vi "ReadBuffer.vi"(2 "Data type":T1(ring)=enum."I16", 5 "Pointer and BufferSize":u64[](array[numeric]), 7 "Offset":u64, 9 "Buffer size":i32, 11 "error in (no error)":errorcluster) -> (6 "Output Array":i16[](array[numeric]), 15 "error out":errorcluster)   [LabVIEW 2020]
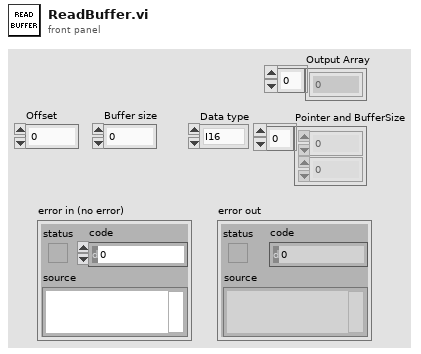
[diagram p1: front panel]
types:
  T1 = enum16{"U8", "I8", "U16", "I16", "U32", "I32", "U64", "I64"}
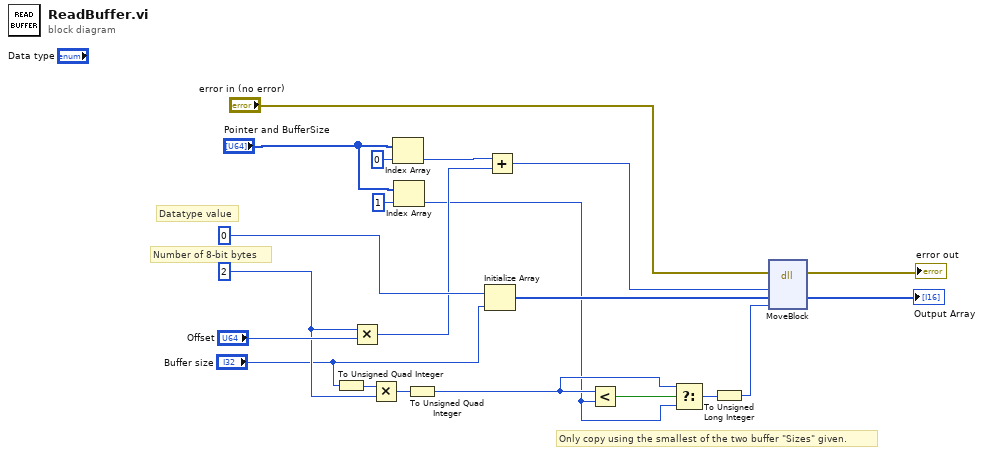
[diagram p0: block diagram]
diagram:
  w6 = u64 2 ("y")
  # "Number of 8-bit bytes"
  # "Datatype value"
  # "Only copy using the smallest of the two buffer \"Sizes\" given."
  n1 = To Unsigned Quad Integer(1:"Buffer size") -> (0:w5:u64)
  n2 = Multiply(x=w6, y="Offset") -> (x*y=w15:u64)
  n3 = Multiply(x=w5, y=w6) -> (x*y=w14:u64)
  n4 = Index Array(array="Pointer and BufferSize", index=0) -> (element=w17:u64)
  n5 = Index Array(array="Pointer and BufferSize", index=1) -> (element=w1:u64)
  n6 = To Unsigned Quad Integer(1:w14) -> (0:w8:u64)
  n7 = Initialize Array(i16 0 ("element"), "Buffer size") -> (w11:i16[])
  n8 = Add(x=w17, y=w15) -> (x+y=w12:u64)
  n9 = Less?(x=w8, y=w1) -> (x < y?=w7:bool)
  n10 = Select(t=w8, s=w7, f=w1) -> (s? t:f=w3:u64)
  n11 = To Unsigned Long Integer(number=w3) -> (unsigned 32bit integer=w2:u32)
  n12 = dll-call lib="LabVIEW" fn="MoveBlock"(error in="error in (no error)", "Source"=w12, "Destination"=w11, "Size"=w2) -> (error out=→"error out":errorcluster, "Destination"=→"Output Array":i16[])  [unwired: 5 in, 1 out]
